vi "Destroy User Events.vi"(11 "UI Template in":refnum<class "UIActorTop.lvclass">) -> (3 "UI Template out":refnum<class "UIActorTop.lvclass">)   [LabVIEW 2021]
uses:
  <userlib>/John_Lib/AbstractActorTemplate/AbstractActorTemplate/UIActorTop.lvclass
  <userlib>/John_Lib/AbstractActorTemplate/AbstractActorTemplate/UIActorTop.lvclass/UIActorTop.ctl
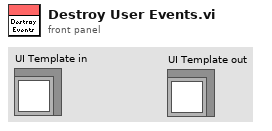
[diagram p1: front panel]
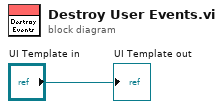
[diagram p0: block diagram]
diagram:
  "UI Template out" <- "UI Template in"
